vi "Create and Send Message Queue.vi"(8 "error in":errorcluster) -> (0 "error out":errorcluster, 3 "queue out":refnum<queue>)   [LabVIEW 2010, in "Visualizer.lvlib"]
uses:
  Visualizer.lvlib
  Message.ctl
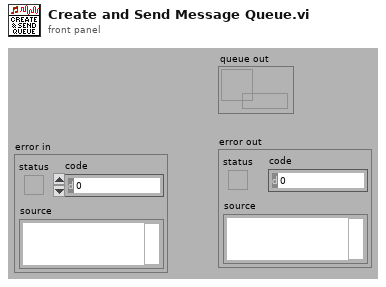
[diagram p1: front panel]
types:
  T1 = typedef "Visualizer.lvlib/Message.ctl" = cluster{"Command":string, "Data":variant}
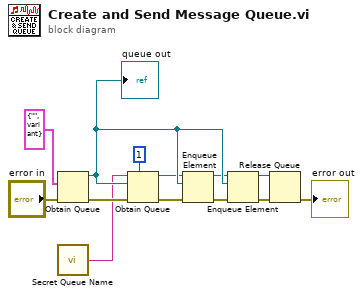
[diagram p0: block diagram]
diagram:
  n1 = Obtain Queue(element data type=T1 {"Command"="", "Data"=variant} ("Message"), error in (no error)="error in") -> (queue out=w12:refnum<queue>, error out=w8:errorcluster)  [unwired: 3 in, 1 out]
  "queue out" <- w12
  n2 = call "Secret Queue Name.vi"() -> ("name (unnamed)"=w2:string)
  n3 = Obtain Queue(max queue size (-1, unlimited)=1, name (unnamed)=w2, element data type=w12, error in (no error)=w8) -> (queue out=w3:refnum<queue>, error out=w5:errorcluster)  [unwired: 1 in, 1 out]
  n4 = Enqueue Element(queue=w3, element=w12, error in (no error)=w5) -> (queue out=w7:refnum<queue>, error out=w6:errorcluster)  [unwired: 1 in, 1 out]
  n5 = Enqueue Element(queue=w7, element=w12, error in (no error)=w6) -> (queue out=w10:refnum<queue>, error out=w11:errorcluster)  [unwired: 1 in, 1 out]
  n6 = Release Queue(queue=w10, error in (no error)=w11) -> (error out=→"error out":errorcluster)  [unwired: 1 in, 2 out]
